vi "Class to Variant.vi"(8 "error in (no error)":errorcluster, 10 "Data in":variant, 11 "CI Project in":refnum<class "CI Project.lvclass">) -> (0 "error out":errorcluster, 1 "Serialized Object Name":string, 2 "Data Out":variant, 3 "CI Project out":refnum<class "CI Project.lvclass">)   [LabVIEW 2014, in "CI Project.lvclass"]
uses:
  CI Project.lvclass
  CI Project.lvclass/CI Project.ctl
  Build Job/Build Job.lvclass
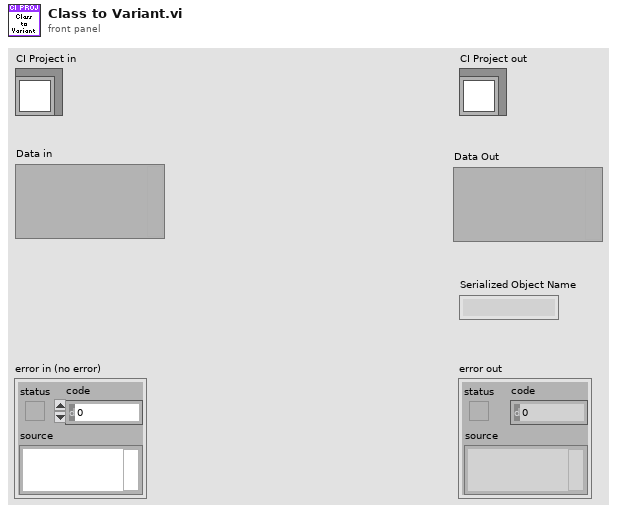
[diagram p1: front panel]
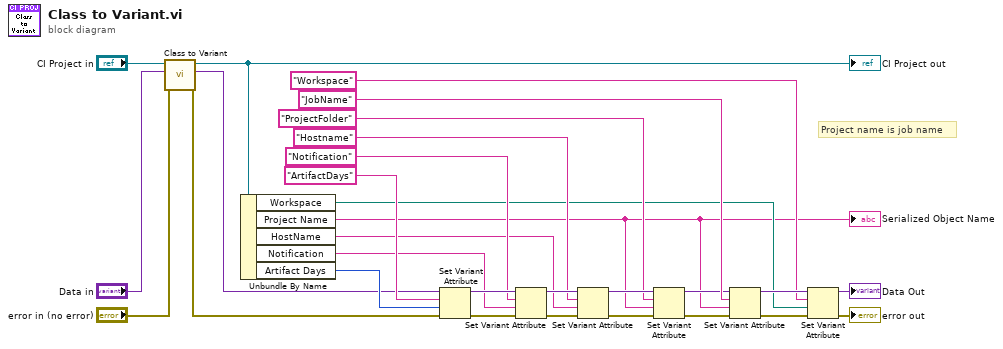
[diagram p0: block diagram]
diagram:
  # "Project name is job name"
  n1 = call-parent "Class to Variant.vi"("error in (no error)"="error in (no error)", "Data in"="Data in", "Build Job in"="CI Project in") -> ("error out"=w12:errorcluster, "Data Out"=w11:variant, "Build Job out"=w15:refnum<class "CI Project.lvclass">)  [unwired: 5 in, 1 out]
  "CI Project out" <- w15
  n2 = Unbundle By Name(w15) -> ("Workspace"=w2:path, "Project Name"=w1:string, "HostName"=w22:string, "Notification"=w23:string, "Artifact Days"=w26:i32)
  "Serialized Object Name" <- w1
  n3 = Set Variant Attribute(Variant=w11, name="ArtifactDays", value=w26, error in=w12) -> (Variant out=w29:variant, error out=w18:errorcluster)  [unwired: 1 out]
  n4 = Set Variant Attribute(Variant=w29, name="Notification", value=w23, error in=w18) -> (Variant out=w28:variant, error out=w17:errorcluster)  [unwired: 1 out]
  n5 = Set Variant Attribute(Variant=w28, name="Hostname", value=w22, error in=w17) -> (Variant out=w27:variant, error out=w16:errorcluster)  [unwired: 1 out]
  n6 = Set Variant Attribute(Variant=w27, name="ProjectFolder", value=w1, error in=w16) -> (Variant out=w7:variant, error out=w9:errorcluster)  [unwired: 1 out]
  n7 = Set Variant Attribute(Variant=w7, name="JobName", value=w1, error in=w9) -> (Variant out=w5:variant, error out=w8:errorcluster)  [unwired: 1 out]
  n8 = Set Variant Attribute(Variant=w5, name="Workspace", value=w2, error in=w8) -> (Variant out=→"Data Out":variant, error out=→"error out":errorcluster)  [unwired: 1 out]
